vi "Launch RT VI.vi"(7 "type specifier VI Refnum (for type only)":refnum<vi>, 8 "error in":errorcluster, 10 "Retries (3)":i32=3, 11 "name (unnamed)":string) -> (0 "error out":errorcluster)   [LabVIEW 2011]
doc: "Launches a VI on a remote RT target.\n\n\nVersion 1.0 - 02/13/2013\n\nPhaeron, Inc.\nwww.phaeron.com\ninfo@phaeron.com"
uses:
  Logger/Log Type.ctl
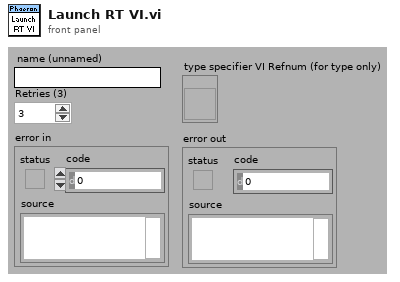
[diagram p1: front panel]
types:
  T1 = typedef "Log Type.ctl" = enum16{"System", "Data", "Error"}
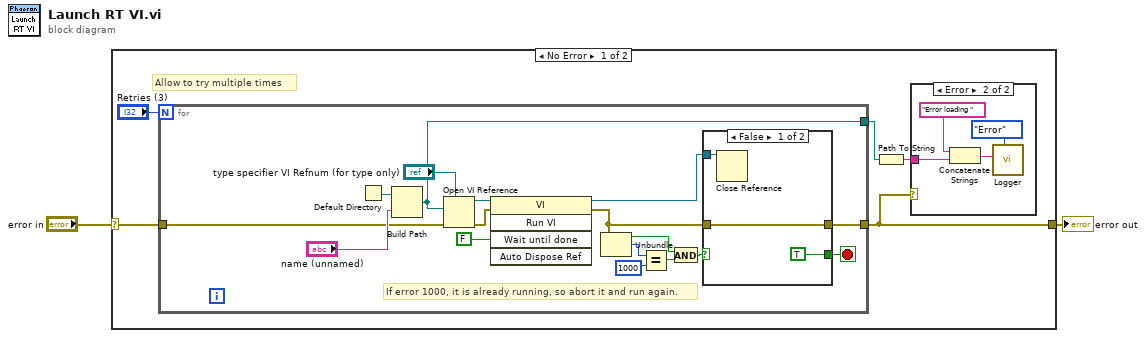
[diagram p0: block diagram]
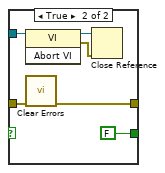
[diagram p3: hidden frame]
diagram:
  n1 = case shown="No Error" "error in" {
    selector: "error in" -> [w7 w38]
    tunnel: [w3 w38] -> w1
    frame No Error {
      # "Allow to try multiple times"
      n2 = for {
        N: "Retries (3)" -> [_]
        tunnel: [w17] -> w3
        tunnel: w7 -> [w16]
        tunnel: [w14] -> w4
        stop <- w15 stop-if-true
        # "If error 1000, it is already running, so abort it and run again."
        n3 = Default Directory() -> (w12:path)
        n4 = Build Path(base path=w12, name or relative path="name (unnamed)") -> (appended path=w14:path)
        n5 = Open VI Reference(type specifier VI Refnum (for type only)="type specifier VI Refnum (for type only)", vi path=w14, error in (no error)=w16) -> (vi reference=w26:refnum<vi>, error out=w27:errorcluster)  [unwired: 3 in]
        n6 = invoke class="VI" method="Run VI"(reference=w26, error in=w27, "Wait until done"=FALSE ("Wait Until Done")) -> (reference out=w18:refnum<vi>, error out=w19:errorcluster)  [unwired: 2 in, 3 out]
        n7 = Unbundle(w19) -> ("status"=w21:bool, "code"=w24:i32)  [unwired: 1 out]
        n8 = Equal?(x=w24, y=1000) -> (x = y?=w22:bool)
        n9 = And(x=w21, y=w22) -> (x .and. y?=w20:bool)
        n10 = case shown="False" w20 {
          tunnel: w19 -> [w30 w37]
          tunnel: [w30 w33] -> w17
          tunnel: w18 -> [w31 w36]
          tunnel: [TRUE FALSE] -> w15
          frame False {
            n11 = Close Reference(reference=w31) -> ()  [unwired: 1 in, 1 out]
          }
          frame True {
            n12 = invoke class="VI" method="Abort VI"(reference=w36) -> (reference out=w34:refnum<vi>, error out=w35:errorcluster)  [unwired: 2 in, 1 out]
            n13 = call <vilib>:"Clear Errors.vi"("error in (no error)"=w37) -> ("error out"=w33:errorcluster)  [unwired: 6 in]
            n14 = Close Reference(reference=w34, error in (no error)=w35) -> ()  [unwired: 1 out]
          }
        }
      }
      n15 = Path To String(path=w4) -> (string=w5:string)
      n16 = case shown="Error" w3 {
        tunnel: w5 -> [_ w9]
        frame No Error {
        }
        frame Error {
          n17 = Concatenate Strings("Error loading " ("regular expression"), w9) -> (w10:string)
          n18 = call "Logger.vi"("Log Type (System)"=Log_Type."Error", "Information"=w10) -> ()  [unwired: 6 in, 4 out]
        }
      }
    }
    frame Error {
    }
  }
  "error out" <- w1
